vi "Robot Global Data.vi"() -> ()   [LabVIEW 2012]
doc: "This global VI can contain as many global variables as you need. Place a control on the panel, give it a good name. To read or write to it from a VI, drag the icon to the diagram of that VI. You can also drag from the project. Click on the node to change which global you access. You shouldn't have multiple locations writing to a global or it will cause a race-condition."
uses:
  <vilib>/Rock Robotics/WPI/Camera/WPI_CameraImageSize.ctl
  <vilib>/Rock Robotics/WPI/DriverStation/WPI_DriverStationRobotMode2.ctl
  <vilib>/Rock Robotics/WPI/Joystick/WPI_JoystickButtonState.ctl
  Auto State Selector.ctl
panel:
  in  "Guess":bool
  in  "Bail Climb":bool
  in  "Climb":bool
  in  "Auto State Selector":T1
  in  "Reset":bool
  out "Shooter Encoder":dbl
  in  "Debug":bool
  out "Left joystick axes":dbl
  out "Right joystick axes":dbl
  in  "Tank Pressure":dbl
  out "Compressor":bool
  out "Auto Debug":bool
  in  "Shooter Clear":bool
  out "Shooter Speed":dbl(knob) scale=0.0..10.0
  in  "Auto-lock":bool
  out "Target Info":T2(array[cluster])
  out "Climber Debug":bool
  out "Shooter Debug":bool
  out "Loader Throttle":dbl
  out "Buttons Joystick":T3
  in  "Shoot":bool
  out "Shooter Throttle":dbl
  in  "High gear":bool
  in  "Tank mode":bool
  out "Right Drive Encoder Rate":dbl
  out "Left Drive Encoder Rate":dbl
  out "Right Joystick Buttons":T3
  out "Left Joystick Buttons":T3
  in  "Robot Mode":T4
  in  "LED toggle rate (ms)":u32=20
  in  "image size":T5=enum."320x240"
  in  "Enable Vision":bool
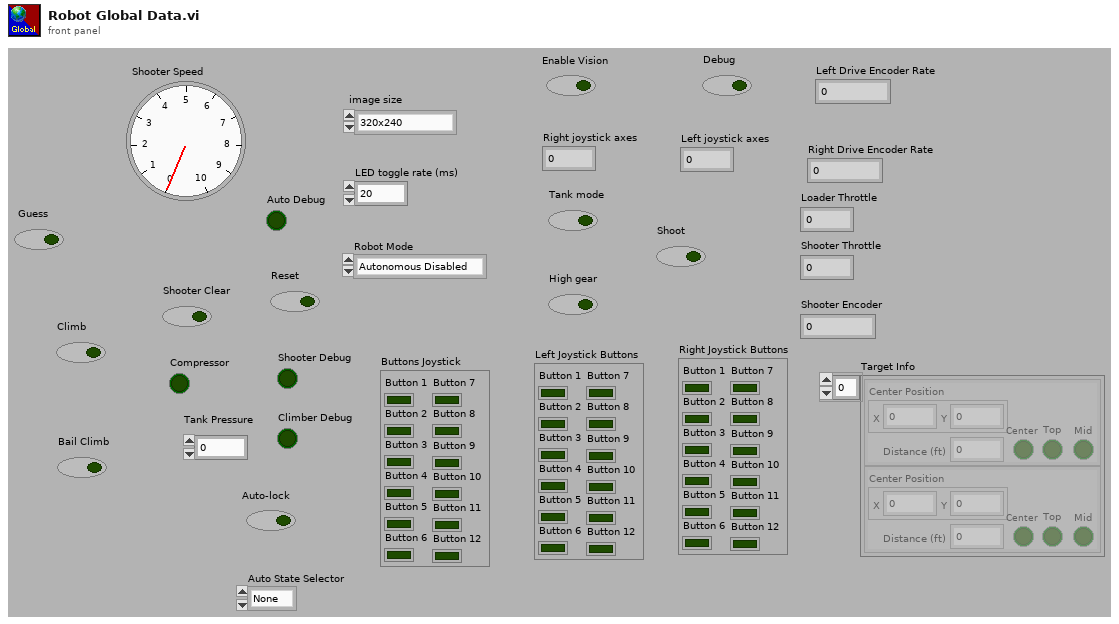
[diagram p1: front panel]
types:
  T1 = typedef "Auto State Selector.ctl" = enum16{"None", "Fire 2x", "Fire 3x", "Dump in low goal"}
  T2 = cluster{"Center Position":cluster{"X":dbl, "Y":dbl}, "Distance (ft)":dbl, "Center":bool, "Top":bool, "Mid":bool}[]
  T3 = typedef "WPI_JoystickButtonState.ctl" = cluster{"Button 1":bool, "Button 2":bool, "Button 3":bool, "Button 4":bool, "Button 5":bool, "Button 6":bool, "Button 7":bool, "Button 8":bool, "Button 9":bool, "Button 10":bool, "Button 11":bool, "Button 12":bool}
  T4 = typedef "WPI_DriverStationRobotMode2.ctl" = enum16{"Autonomous Disabled", "Autonomous Enabled", "Teleop Disabled", "Teleop Enabled", "Timeout", "Finish", "Test Disabled", "Test Enabled"}
  T5 = typedef "WPI_CameraImageSize.ctl" = enum16{"640x480", "320x240", "160x120"}
diagram:
